vi "Write Single Coil1.vi"(8 "error in (no error)":errorcluster, 9 "coil value":bool, 10 "address":u16, 11 "device data model in":refnum<class "Standard Data Model1.lvclass">) -> (0 "error out":errorcluster, 3 "device data model out":refnum<class "Standard Data Model1.lvclass">)   [LabVIEW 2021, in "NI_modbus_upd.lvlib" / "Standard Data Model1.lvclass"]
doc: "Writes the value of a single coil."
uses:
  Standard Data Model1.lvclass
  Standard Data Model1.lvclass/Standard Data Model1.ctl
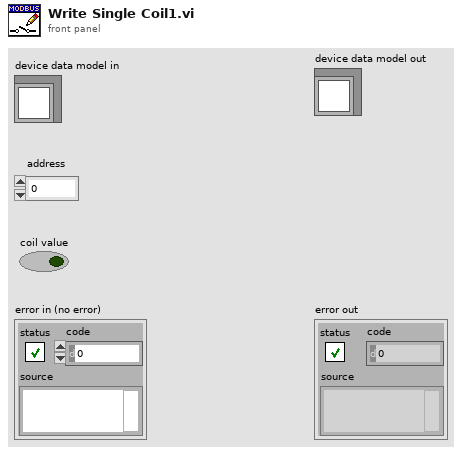
[diagram p1: front panel]
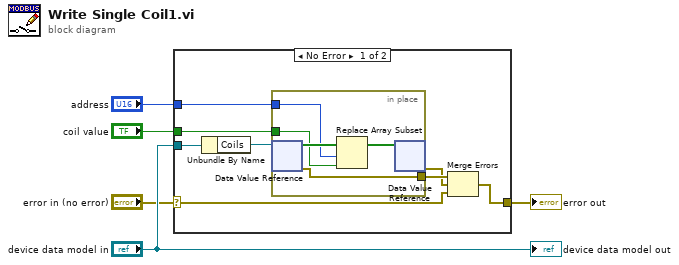
[diagram p0: block diagram]
diagram:
  n1 = case shown="No Error" "error in (no error)" {
    selector: "error in (no error)" -> [w6 w19]
    tunnel: "device data model in" -> [w13 _]
    tunnel: "coil value" -> [w11 _]
    tunnel: [w10 w19] -> w3
    tunnel: "address" -> [w9 _]
    frame No Error {
      n2 = Unbundle By Name(w13) -> ("Coils"=w12:refnum<data-value>)
      n3 = in-place {
        in-place-border: w11 -> [w16]
        in-place-border: w9 -> [w15]
        in-place-border: [w14] -> w8
        n4 = in-place-dvr #1(w12) -> (w18:bool[], w14:errorcluster)
        n5 = Replace Array Subset(array=w18, new element=w16, index=w15) -> (w17:bool[])
        n6 = in-place-dvr #1(w17) -> (w7:errorcluster)  [unwired: 1 out]
      }
      n7 = Merge Errors(w8, w7, w6) -> (w10:errorcluster)
    }
    frame Error {
    }
  }
  "error out" <- w3
  "device data model out" <- "device data model in"
